vi "data-center-monitor-compare-power-rate.vi"() -> ()   [LabVIEW 2024]
doc: "Demonstrates how to implement advanced power measurement of harmonic parameters on a three-phase electrical power system, such as measurement of harmonic distortion factor, total harmonic distortion, harmonic power, etc. Measurement of harmonic parameters is based on a resampling algorithm."
uses:
  <vilib>/Utility/error.llb/DialogType.ctl
  <vilib>/addons/Electrical Power/Power Measurement/subVIs/ep_Resampled Data.ctl
  <vilib>/DAQmx/read.llb/DAQmx Read (Analog 1D Wfm NChan NSamp).vi
  <extravilib>/ChannelInstances/Tag-bool/Read.vi
  <extravilib>/ChannelInstances/Tag-bool/Write With Abort.vi
  <extravilib>/ChannelInstances/Tag-bool/Read With Abort.vi
  <extravilib>/ChannelInstances/Tag-bool/Instantiate.vi
  <extravilib>/ChannelInstances/Tag-bool/EndpointRead.vi
  <extravilib>/ChannelInstances/Tag-bool/Endpoint.vi
  <vilib>/addons/Electrical Power/Basic/Measurement/Fundamental Vector (N Channels).vi
  <vilib>/DAQmx/miscellaneous.llb/DAQmx Fill In Error Info.vi
  <vilib>/DAQmx/create/channels.llb/DAQmx Create Channel (AI-Voltage-Basic).vi
  <vilib>/DAQmx/create/channels.llb/DAQmx Create Channel (AI-Current-Basic).vi
  <vilib>/DAQmx/configure/timing.llb/DAQmx Timing (Sample Clock).vi
  <resource>/objmgr/daqmx.rc
  <vilib>/addons/Electrical Power/Power Measurement/NI_EP_Power Measurement.lvlib
  <vilib>/addons/Electrical Power/Basic/NI_EP_Basic.lvlib
  <extravilib>/ChannelInstances/Tag-bool.lvlib
panel:
  in  "Display":T1(tab)
  in  "Configuration":enum32{"DAQmx", "Others"}(tab)
  in  "number of samples per channel":i32=10000
  in  "DAQmx sample rate [Hz]":dbl=50000.0 format="%0.2f"
  in  "current channels":tag="current-input/ai0:2"
  in  "maximum current value":dbl=0.002 format="%0.3f"
  in  "minimum current value":dbl=-0.002 format="%0.3f"
  in  "voltage channels":tag="voltage-input/ai0:2"
  in  "maximum voltage value":dbl=300.0 format="%0.2f"
  in  "minimum voltage value":dbl=-300.0 format="%0.2f"
  in  "frequency range [Hz]":cluster{"minimum":dbl, "maximum":dbl}={"minimum"=45.0, "maximum"=65.0}
  in  "samples per cycle":u16=192
  in  "cycles per block":u16=10
  in  "maximum harmonic  order":u16=50
  in  "distortion factor denominator":enum16{"Fundamental value", "Total value"}(ring)
  in  "filter for frequency measurement":T2={"enable filter? (T)"=TRUE, "passband edge frequency [Hz]"=65.0, "passband ripple [dB]"=0.1, "stopband edge frequency [Hz]"=85.0, "stopband attenuation [dB]"=60.0}
  out "Service Rack":cluster{dbl[], dbl[]}[](graph)
  out "PDU":cluster{dbl[], dbl[]}[](graph)
  out "V THD [%]":dbl[](array[numeric]) format="%#_2g"
  out "I THD [%]":dbl[](array[numeric]) format="%#_2g"
  out "Average Frequency [Hz]":dbl format="%#_4g"
  out "Power Usage":T3(graph)
  in  "pause wfm":bool
  out "Time Domain":T4(graph)
  in  "Pause Button":bool
  out "Active Power":waveform(dbl)[](graph)
  out "Voltage Harmonic Spectra":T5(graph)
  out "Current Harmonic Spectra":T5(graph)
  out "voltage total values":dbl[](array[numeric])
  out "voltage THD [%]":dbl[](array[numeric])
  out "voltage harmonic distortion factors [%]":dbl[][](array[numeric])
  out "current THD [%]":dbl[](array[numeric])
  out "total power value":T3
  out "harmonic power values":T6(array[cluster])
  out "power values":T7(array[cluster])
  out "Fundamental Voltage Vectors (Vrms)":cluster{dbl[], dbl[]}[](graph)
  out "Fundamental Current Vectors (Arms)":cluster{dbl[], dbl[]}[](graph)
  out "power history":T3(graph)
  in  "pause-update":bool
  in  "stop":bool
  # "Data Center Power Monitor Demo"
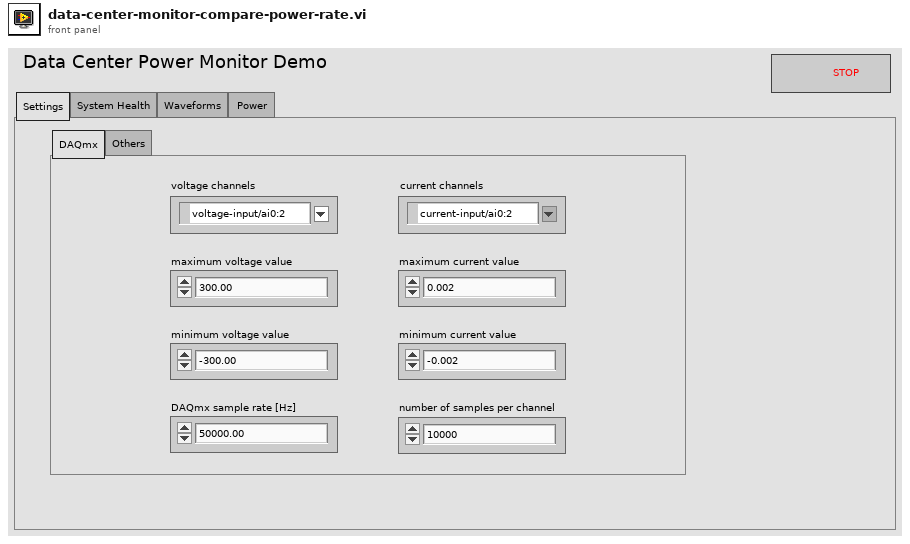
[diagram p1: front panel]
types:
  T1 = enum32{"Settings", "System Health", "Waveforms", "Power ", "V Spectra", "I Spectra", "Basic Parameters", "Harmonic Power", "Phasor", "History"}
  T2 = cluster{"enable filter? (T)":bool, "passband edge frequency [Hz]":dbl, "passband ripple [dB]":dbl, "stopband edge frequency [Hz]":dbl, "stopband attenuation [dB]":dbl}
  T3 = cluster{"active power [W]":dbl, "apparent power [VA]":dbl, "reactive power [VAR]":dbl, "power factor":dbl}
  T4 = cluster{"times [s]":dbl[], "resampled signal":dbl[]}[]
  T5 = cluster{"order 0":dbl, "delta order":dbl, "complex spectrum":dbl[]}[]
  T6 = cluster{"active power [W]":dbl, "apparent power [VA]":dbl, "reactive power [VAR]":dbl, "power factor":dbl}[][]
  T7 = cluster{"active power [W]":dbl, "apparent power [VA]":dbl, "reactive power [VAR]":dbl, "power factor":dbl}[]
  T8 = typedef "NI_EP_Power Measurement.lvlib/ep_Resampled Data.ctl" = cluster{"times [s]":dbl[], "resampled signal":dbl[]}
  T9 = typedef "DialogType.ctl" = u16
  T10 = cluster{"zero crossing times [s]":dbl[], "zero crossings per cycle":u8}
  T11 = typedef "Tag-bool.lvlib/))Channel.ctl" = refnum<queue>
  T12 = cluster{"order 0":dbl, "delta order":dbl, "complex spectrum":cdb[]}[]
  T13 = typedef "NI_EP_Basic.lvlib/basic_Power Value.ctl" = cluster{"active power [W]":dbl, "apparent power [VA]":dbl, "reactive power [VAR]":dbl, "power factor":dbl}
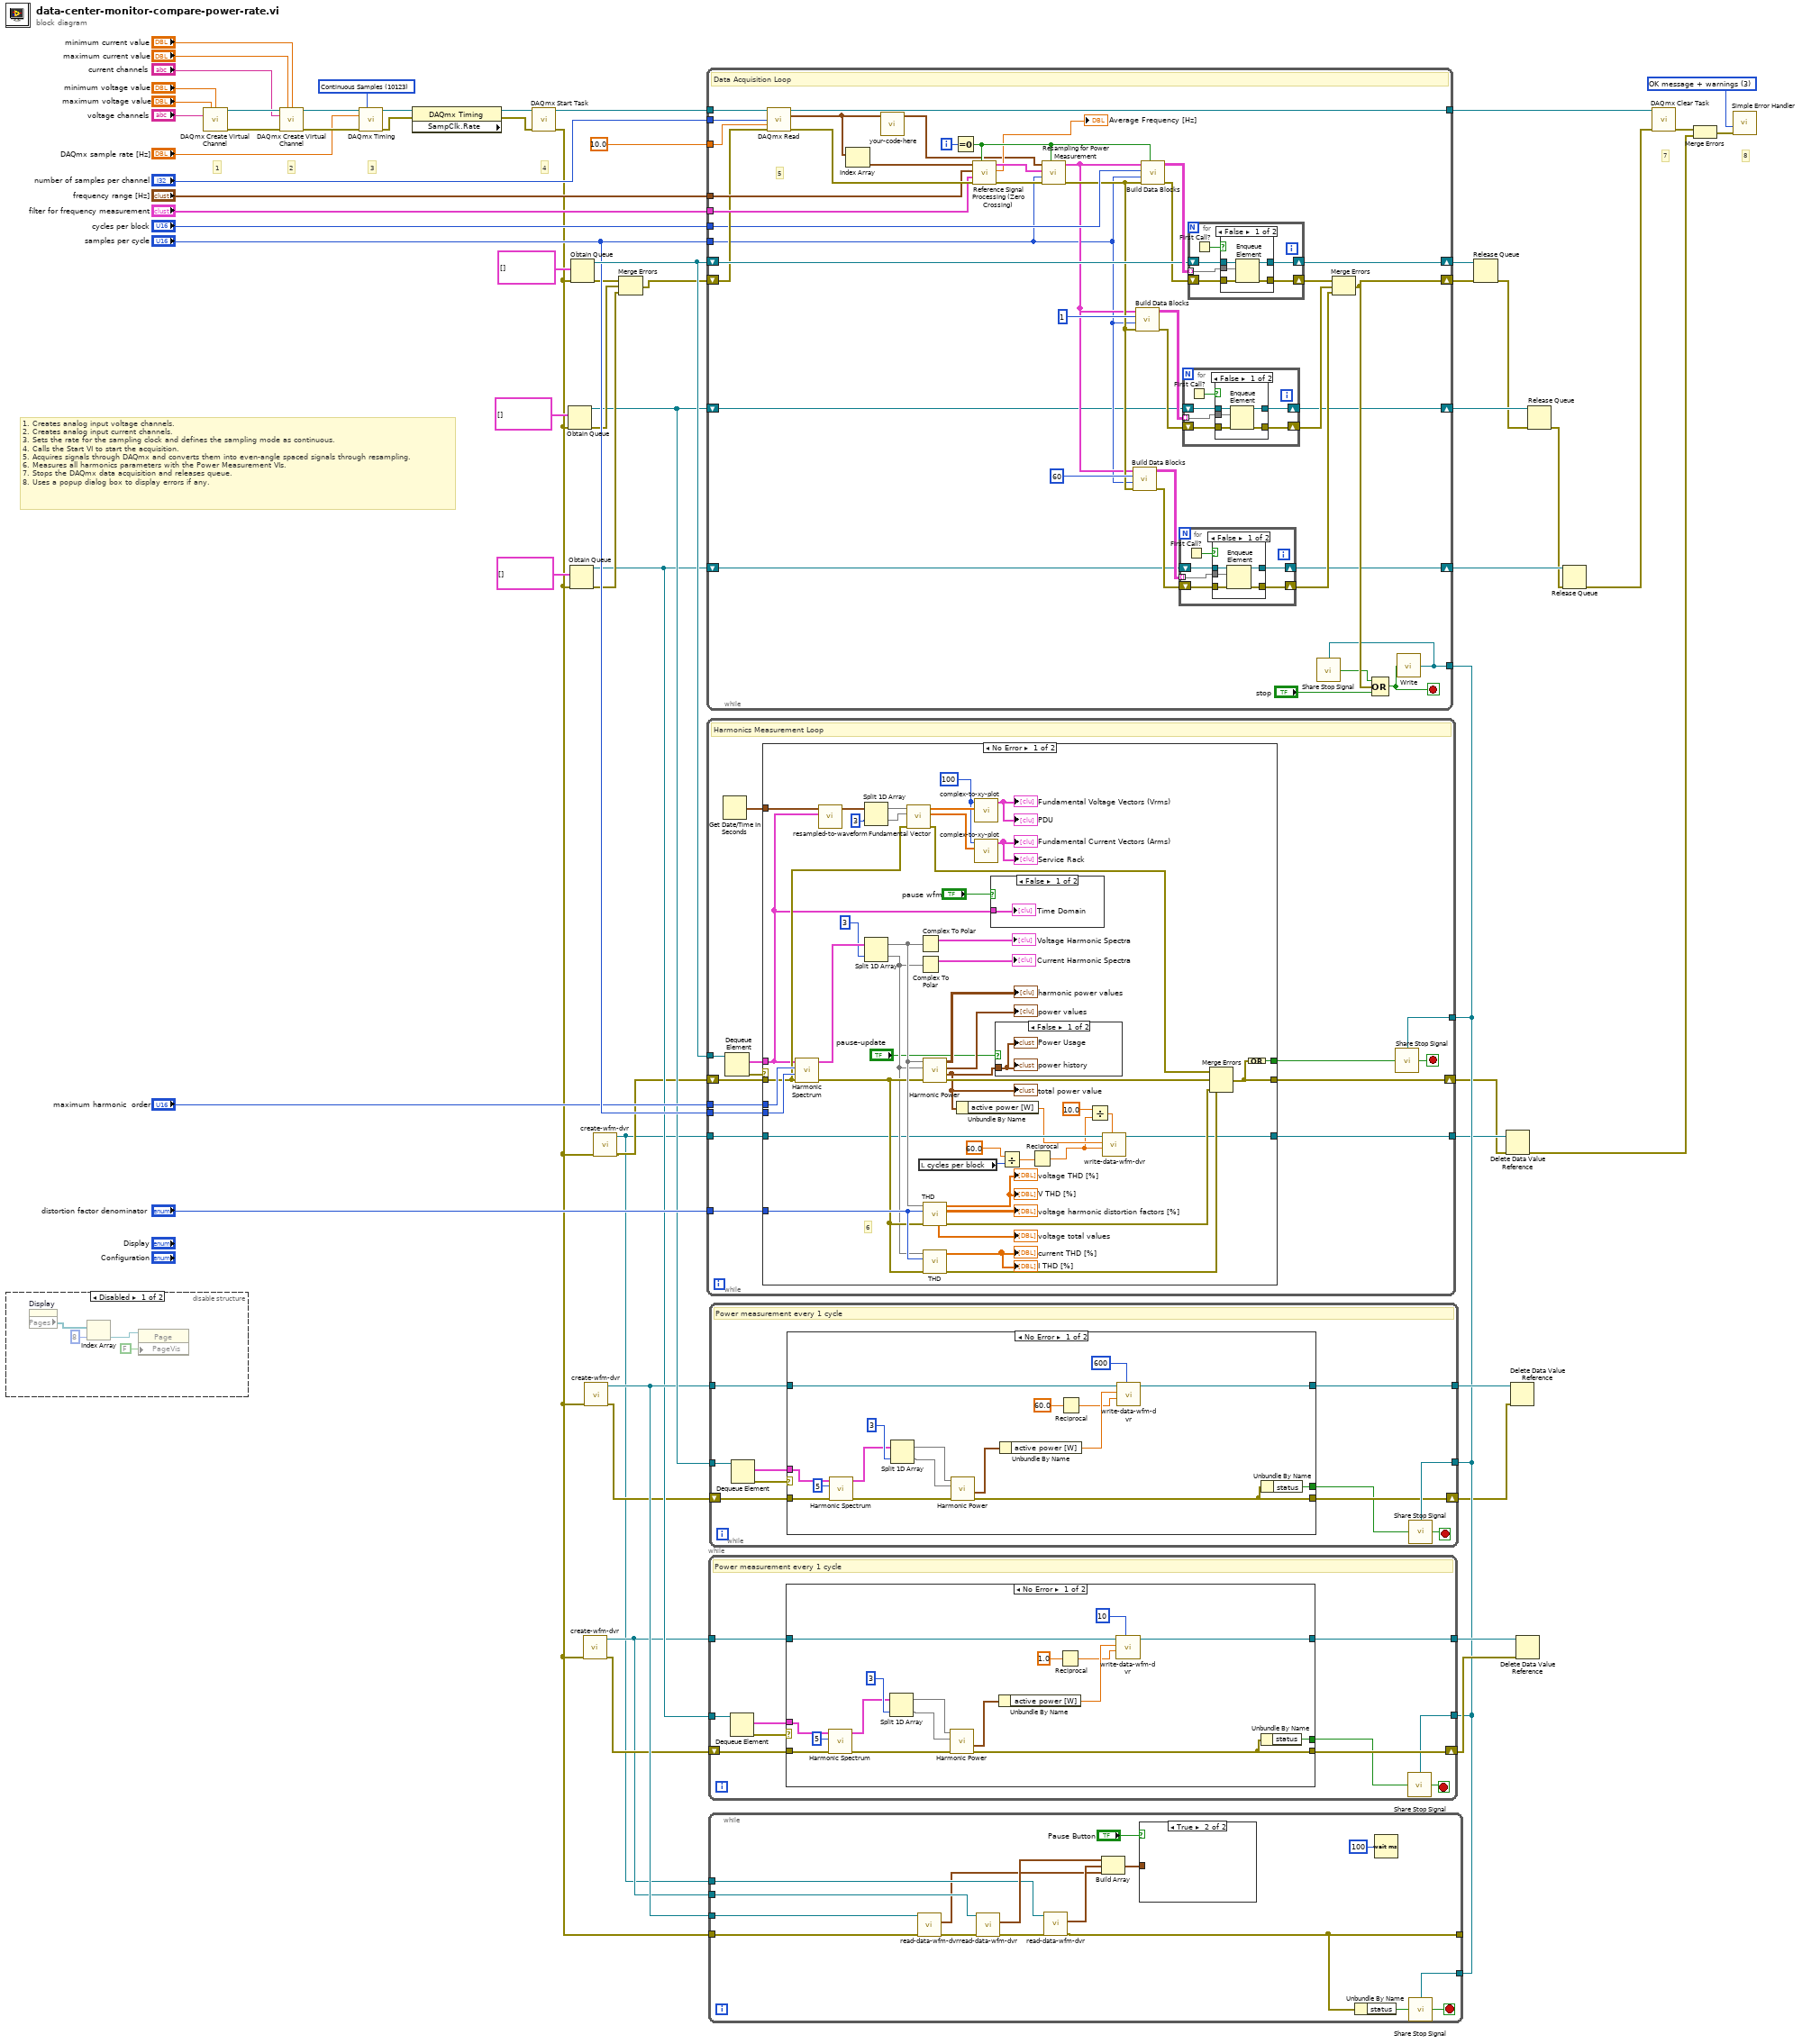
[diagram p0: block diagram]
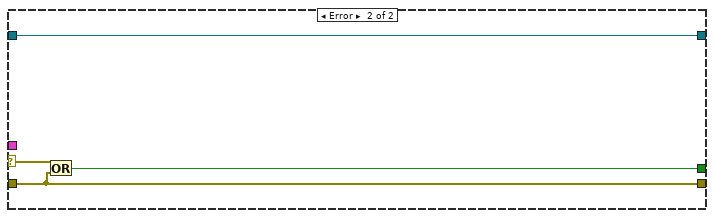
[diagram p3: hidden frame]
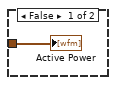
[diagram p4: hidden frame]
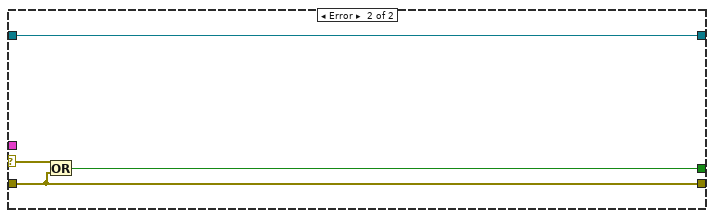
[diagram p5: hidden frame]
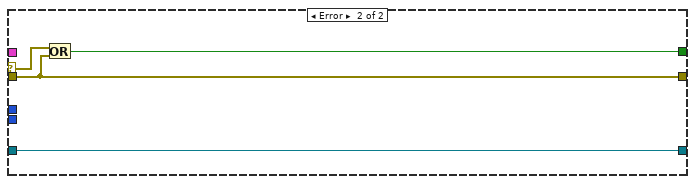
[diagram p8: hidden frame]
diagram:
  w32 = T9 3 items=["no dialog", "OK message", "continue or stop message", "OK message + warnings", "continue/stop + warnings"] ("type of dialog (OK msg:1)")
  w34 = 10123 items=["Finite Samples"=10178, "Continuous Samples"=10123, "Hardware Timed Single Point"=12522] ("sample mode")
  # "8"
  # "7"
  # "1. Creates analog input voltage channels.\n2. Creates analog input current channels.\n3. Sets the rate for the sampling clock and defines the sampling mode as continuous.\n4. Calls the Start VI to start the acquisition.\n5. Acquires signals through DAQmx and converts them into even-angle spaced signals through resampling. \n6. Measures all harmonics parameters with the Power Measurement VIs.\n7.\tStops the DAQmx data acquisition and releases queue.\n8. Uses a popup dialog box to display errors if any."
  # "4"
  # "3"
  # "2"
  # "1"
  n1 = disable-structure shown="Disabled" {
    frame Disabled {
      n2 = property on="Display" class="TabCtl (strict)"() -> ("Pages"=w65:refnum<vi>[])  [unwired: 2 in, 2 out]
      n3 = Index Array(array=w65, index=8) -> (element=w64:refnum<vi>)
      n4 = property class="Page"(reference=w64, "PageVis"=FALSE ("Page Visible")) -> ()  [unwired: 1 in, 2 out]
    }
    frame Enabled {
    }
  }
  n5 = call-poly <vilib>:"DAQmx Create Virtual Channel.vi"("maximum value"="maximum voltage value", "minimum value"="minimum voltage value", "physical channels"="voltage channels") -> ("task out"=w57:refnum<k21>, "error out"=w58:errorcluster)  [unwired: 11 in]
  n6 = call-poly <vilib>:"DAQmx Create Virtual Channel.vi"("task in"=w57, "maximum value"="maximum current value", "minimum value"="minimum current value", "physical channels"="current channels", "error in"=w58) -> ("task out"=w52:refnum<k21>, "error out"=w53:errorcluster)  [unwired: 9 in]
  n7 = call-poly <vilib>:"DAQmx Timing.vi"("task/channels in"=w52, "sample mode"=w34, "rate"="DAQmx sample rate [Hz]", "error in"=w53) -> ("task out"=w46:refnum<k21>, "error out"=w50:errorcluster)  [unwired: 10 in]
  n8 = property class="DAQmx Timing" props=["SampClk.Rate"](reference=w46, error in=w50) -> (reference out=w49:refnum<k21>, error out=w48:errorcluster)  [unwired: 1 out]
  n9 = call <vilib>:"DAQmx Start Task.vi"("task/channels in"=w49, "error in"=w48) -> ("task out"=w47:refnum<k21>, "error out"=w6:errorcluster)  [unwired: 12 in]
  n10 = Obtain Queue(element data type=T8[] [] ("resampled data"), error in (no error)=w6) -> (queue out=w17:refnum<queue>, error out=w24:errorcluster)  [unwired: 3 in, 1 out]
  n11 = Obtain Queue(element data type=T8[] [] ("resampled data"), error in (no error)=w6) -> (queue out=w14:refnum<queue>, error out=w23:errorcluster)  [unwired: 3 in, 1 out]
  n12 = Obtain Queue(element data type=T8[] [] ("resampled data"), error in (no error)=w6) -> (queue out=w39:refnum<queue>, error out=w26:errorcluster)  [unwired: 3 in, 1 out]
  n13 = call "create-wfm-dvr.vi"("error in (no error)"=w6) -> ("error out"=w12:errorcluster, "wfm dvr"=w11:refnum<data-value>)  [unwired: 9 in]
  n14 = call "create-wfm-dvr.vi"("error in (no error)"=w6) -> ("error out"=w13:errorcluster, "wfm dvr"=w15:refnum<data-value>)  [unwired: 9 in]
  n15 = call "create-wfm-dvr.vi"("error in (no error)"=w6) -> ("error out"=w5:errorcluster, "wfm dvr"=w1:refnum<data-value>)  [unwired: 9 in]
  n16 = Merge Errors(w26, w24, w23) -> (w25:errorcluster)
  n17 = while {
    tunnel: "number of samples per channel" -> [w106]
    tunnel: w47 -> [w107]
    tunnel: [w105] -> w44
    tunnel: "frequency range [Hz]" -> [w101]
    tunnel: "filter for frequency measurement" -> [w100]
    shift-right: [w93] -> w41
    shift-left: w39 -> [w95]
    shift-right: [w75] -> w30
    shift-left: w25 -> [w94]
    tunnel: "samples per cycle" -> [w77]
    tunnel: "cycles per block" -> [w92]
    tunnel: 10.0 ("timeout") -> [w90]
    shift-right: [w71] -> w22
    shift-left: w17 -> [w72]
    shift-right: [w69] -> w20
    shift-left: w14 -> [w70]
    tunnel: [w67] -> w8
    i -> [w103]
    stop <- w68 stop-if-true
    # "5"
    # "Data Acquisition Loop"
    n18 = call-poly <vilib>:"DAQmx Read.vi"("task/channels in"=w107, "number of samples per channel"=w106, "timeout"=w90, "error in"=w94) -> ("task out"=w105:refnum<k21>, "data"=w87:waveform(dbl)[], "error out"=w104:errorcluster)  [unwired: 9 in]
    n19 = Index Array(array=w87) -> (element=w102:waveform(dbl))  [unwired: 1 in]
    n20 = call "your-code-here.vi"("data in"=w87) -> ("data out"=w86:waveform(dbl)[])  [unwired: 10 in]
    n21 = Equal To 0?(x=w103) -> (x = 0?=w97:bool)
    n22 = call <vilib>:"Reference Signal Processing (Zero Crossing).vi"("reset? (F)"=w97, "error in (no error)"=w104, "filter for frequency measurement"=w100, "frequency range [Hz]"=w101, "reference signal"=w102) -> ("error out"=w99:errorcluster, "average frequency [Hz]"=→"Average Frequency [Hz]":dbl, "zero crossing information"=w98:T10)  [unwired: 3 in, 1 out]
    n23 = call <vilib>:"Resampling for Power Measurement.vi"("reset? (F)"=w97, "error in (no error)"=w99, "samples per cycle (192)"=w77, "trigger information"=w98, "data in"=w86) -> ("error out"=w79:errorcluster, "resampled data"=w78:T8[])  [unwired: 5 in]
    n24 = call <vilib>:"Build Data Blocks.vi"("error in (no error)"=w79, "samples per cycle (192)"=w77, "cycles per block (10)"=u16 60, "resampled data"=w78) -> ("error out"=w81:errorcluster, "data blocks"=w80:T8[][])  [unwired: 6 in]
    n25 = call <vilib>:"Build Data Blocks.vi"("error in (no error)"=w79, "samples per cycle (192)"=w77, "cycles per block (10)"=u16 1, "resampled data"=w78) -> ("error out"=w84:errorcluster, "data blocks"=w85:T8[][])  [unwired: 6 in]
    n26 = call <vilib>:"Build Data Blocks.vi"("reset? (F)"=w97, "error in (no error)"=w79, "samples per cycle (192)"=w77, "cycles per block (10)"=w92, "resampled data"=w78) -> ("error out"=w89:errorcluster, "data blocks"=w96:T8[][])  [unwired: 5 in]
    n27 = for {
      shift-right: [w111] -> w69
      shift-left: w70 -> [w112]
      shift-right: [w113] -> w73
      shift-left: w81 -> [w110]
      tunnel: w80 -> [w109] mode=indexing
      n28 = First Call?() -> (First Call?: T/F=w108:bool)
      n29 = case shown="False" w108 {
        tunnel: [w118 w119] -> w113
        tunnel: w112 -> [w117 w120]
        tunnel: [w116 w120] -> w111
        tunnel: w110 -> [w115 w119]
        tunnel: w109 -> [w114 _]
        frame False {
          n30 = Enqueue Element(queue=w117, element=w114, error in (no error)=w115) -> (queue out=w116:refnum<queue>, error out=w118:errorcluster)  [unwired: 1 in, 1 out]
        }
        frame True {
        }
      }
    }
    n31 = for {
      shift-right: [w124] -> w71
      shift-left: w72 -> [w125]
      shift-right: [w126] -> w74
      shift-left: w84 -> [w123]
      tunnel: w85 -> [w122] mode=indexing
      n32 = First Call?() -> (First Call?: T/F=w121:bool)
      n33 = case shown="False" w121 {
        tunnel: [w131 w132] -> w126
        tunnel: w125 -> [w130 w133]
        tunnel: [w129 w133] -> w124
        tunnel: w123 -> [w128 w132]
        tunnel: w122 -> [w127 _]
        frame False {
          n34 = Enqueue Element(queue=w130, element=w127, error in (no error)=w128) -> (queue out=w129:refnum<queue>, error out=w131:errorcluster)  [unwired: 1 in, 1 out]
        }
        frame True {
        }
      }
    }
    n35 = for {
      shift-right: [w137] -> w93
      shift-left: w95 -> [w138]
      shift-right: [w139] -> w76
      shift-left: w89 -> [w136]
      tunnel: w96 -> [w135] mode=indexing
      n36 = First Call?() -> (First Call?: T/F=w134:bool)
      n37 = case shown="False" w134 {
        tunnel: [w144 w145] -> w139
        tunnel: w138 -> [w143 w146]
        tunnel: [w142 w146] -> w137
        tunnel: w136 -> [w141 w145]
        tunnel: w135 -> [w140 _]
        frame False {
          n38 = Enqueue Element(queue=w143, element=w140, error in (no error)=w141) -> (queue out=w142:refnum<queue>, error out=w144:errorcluster)  [unwired: 1 in, 1 out]
        }
        frame True {
        }
      }
    }
    n39 = Merge Errors(w76, w74, w73) -> (w75:errorcluster)
    n40 = call <vilib>:"Share Stop Signal.vi"("channel"=w67) -> ("stop"=w66:bool)  [unwired: 1 in]
    n41 = Compound Arithmetic op=OR(w66, w75, "stop") -> (w68:bool)
    n42 = call <extravilib>:"Write.vi"("element"=w68) -> ("channel"=w67:T11)  [unwired: 1 out]
  }
  n43 = while {
    shift-right: [w152] -> w3
    shift-left: w5 -> [w155]
    tunnel: w39 -> [w160]
    tunnel: "samples per cycle" -> [w158]
    tunnel: "maximum harmonic  order" -> [w157]
    tunnel: "distortion factor denominator" -> [w156]
    tunnel: w8 -> [w149]
    tunnel: w1 -> [w148]
    tunnel: [w147] -> w4
    stop <- w153 stop-if-true
    # "Harmonics Measurement Loop"
    n44 = Get Date/Time In Seconds() -> (seconds since 1Jan1904=w150:timestamp)
    n45 = Dequeue Element(queue=w160) -> (element=w159:T8[], error out=w154:errorcluster)  [unwired: 2 in, 2 out]
    n46 = case shown="No Error" w154 {
      selector: w154 -> [_ w212]
      tunnel: w159 -> [w165 _]
      tunnel: w158 -> [w206 _]
      tunnel: w157 -> [w205 _]
      tunnel: w155 -> [w183 w211]
      tunnel: [w198 w211] -> w152
      tunnel: w156 -> [w202 _]
      tunnel: [w193 w210] -> w151
      tunnel: w150 -> [w191 _]
      tunnel: w148 -> [w174 w209]
      tunnel: [w173 w209] -> w147
      frame No Error {
        w184 = 100
        # "6"
        n47 = call <vilib>:"Harmonic Spectrum.vi"("error in (no error)"=w183, "samples per cycle (192)"=w206, "maximum harmonic order (50)"=w205, "resampled data"=w165) -> ("error out"=w194:errorcluster, "harmonic spectra"=w204:T12)  [unwired: 6 in]
        n48 = call "resampled-to-waveform.vi"("resampled data"=w165, "current-timestamp"=w191) -> ("waveform data"=w189:waveform(dbl)[])  [unwired: 9 in]
        n49 = Split 1D Array(array=w189, index=3) -> (first subarray=w188:waveform(dbl)[], second subarray=w187:waveform(dbl)[])
        n50 = Split 1D Array(array=w204, index=3) -> (first subarray=w203:T12, second subarray=w180:T12)
        n51 = call-poly <vilib>:"Fundamental Vector.vi"("error in (no error)"=w183, "current waveforms"=w187, "voltage waveforms"=w188) -> ("error out"=w182:errorcluster, "current fundamental vectors"=w185:cdb[], "voltage fundamental vectors"=w186:cdb[])  [unwired: 5 in, 1 out]
        n52 = Complex To Polar(r * e^(i*theta)=w203) -> (r=→"Voltage Harmonic Spectra":T5)  [unwired: 1 out]
        n53 = Complex To Polar(r * e^(i*theta)=w180) -> (r=→"Current Harmonic Spectra":T5)  [unwired: 1 out]
        n54 = local read "cycles per block"() -> (w171:u16)
        n55 = call <vilib>:"Harmonic Power.vi"("error in (no error)"=w194, "current spectra"=w180, "voltage spectra"=w203) -> ("error out"=w199:errorcluster, "total power value"=w162:T13, "power values"=→"power values":T13[], "harmonic power values"=→"harmonic power values":T13[][])  [unwired: 5 in]
        "total power value" <- w162
        n56 = call <vilib>:"THD.vi"("error in (no error)"=w194, "distortion factor denominator"=w202, "harmonic spectra"=w203) -> ("error out"=w195:errorcluster, "harmonic distortion factors [%]"=→"voltage harmonic distortion factors [%]":dbl[][], "THD [%]"=→"voltage THD [%]" →"V THD [%]":dbl[], "total values"=→"voltage total values":dbl[])  [unwired: 5 in]
        n57 = call <vilib>:"THD.vi"("error in (no error)"=w194, "distortion factor denominator"=w202, "harmonic spectra"=w180) -> ("error out"=w197:errorcluster, "THD [%]"=→"current THD [%]" →"I THD [%]":dbl[])  [unwired: 5 in, 2 out]
        n58 = Unbundle By Name(w162) -> ("active power [W]"=w172:dbl)
        n59 = call "complex-to-xy-plot.vi"("complex-vector"=w186, "number-of-points"=w184) -> ("xy-plot-output"=→"Fundamental Voltage Vectors (Vrms)" →"PDU":cluster{dbl[], dbl[]}[])  [unwired: 9 in]
        n60 = call "complex-to-xy-plot.vi"("complex-vector"=w185, "number-of-points"=w184) -> ("xy-plot-output"=→"Fundamental Current Vectors (Arms)" →"Service Rack":cluster{dbl[], dbl[]}[])  [unwired: 9 in]
        n61 = case shown="False" "pause wfm" {
          tunnel: w165 -> [w207 _]
          frame False {
            "Time Domain" <- w207
          }
          frame True {
          }
        }
        n62 = case shown="False" "pause-update" {
          tunnel: w162 -> [w208 _]
          frame False {
            "power history" <- w208
            "Power Usage" <- w208
          }
          frame True {
          }
        }
        n63 = Divide(x=60.0, y=w171) -> (x/y=w169:dbl)
        n64 = Reciprocal(x=w169) -> (1/x=w167:dbl)
        n65 = Divide(x=10.0, y=w167) -> (x/y=w166:dbl)
        n66 = call "write-data-wfm-dvr.vi"("wfm size"=w166, "dt"=w167, "data"=w172, "wfm dvr"=w174) -> ("wfm dvr"=w173:refnum<data-value>)  [unwired: 6 in, 1 out]
        n67 = Merge Errors(w182, w199, w195, w197) -> (w198:errorcluster)
        n68 = Compound Arithmetic op=OR(w198) -> (w193:bool)
      }
      frame Error {
        n69 = Or(x=w212, y=w211) -> (x .or. y?=w210:bool)
      }
    }
    n70 = call <vilib>:"Share Stop Signal.vi"("set stop (F)"=w151, "channel"=w149) -> ("stop"=w153:bool)
  }
  n71 = while {
    shift-right: [w217] -> w9
    shift-left: w12 -> [w221]
    tunnel: w14 -> [w222]
    tunnel: w8 -> [w213]
    tunnel: w11 -> [w215]
    tunnel: [w214] -> w10
    stop <- w218 stop-if-true
    # "Power measurement every 1 cycle"
    n72 = Dequeue Element(queue=w222) -> (element=w219:T8[], error out=w220:errorcluster)  [unwired: 2 in, 2 out]
    n73 = case shown="No Error" w220 {
      selector: w220 -> [_ w243]
      tunnel: w221 -> [w238 w242]
      tunnel: w219 -> [w235 _]
      tunnel: [w228 w242] -> w217
      tunnel: [w239 w241] -> w216
      tunnel: w215 -> [w227 w240]
      tunnel: [w226 w240] -> w214
      frame No Error {
        n74 = call <vilib>:"Harmonic Spectrum.vi"("error in (no error)"=w238, "maximum harmonic order (50)"=u16 5, "resampled data"=w235) -> ("error out"=w234:errorcluster, "harmonic spectra"=w236:T12)  [unwired: 7 in]
        n75 = Split 1D Array(array=w236, index=3) -> (first subarray=w233:T12, second subarray=w232:T12)
        n76 = call <vilib>:"Harmonic Power.vi"("error in (no error)"=w234, "current spectra"=w232, "voltage spectra"=w233) -> ("error out"=w228:errorcluster, "total power value"=w231:T13)  [unwired: 5 in, 2 out]
        n77 = Unbundle By Name(w231) -> ("active power [W]"=w225:dbl)
        n78 = Reciprocal(x=1.0) -> (1/x=w224:dbl)
        n79 = call "write-data-wfm-dvr.vi"("wfm size"=10, "dt"=w224, "data"=w225, "wfm dvr"=w227) -> ("wfm dvr"=w226:refnum<data-value>)  [unwired: 6 in, 1 out]
        n80 = Unbundle By Name(w228) -> ("status"=w239:bool)
      }
      frame Error {
        n81 = Or(x=w243, y=w242) -> (x .or. y?=w241:bool)
      }
    }
    n82 = call <vilib>:"Share Stop Signal.vi"("set stop (F)"=w216, "channel"=w213) -> ("stop"=w218:bool)
  }
  n83 = while {
    tunnel: w6 -> [w256]
    tunnel: w8 -> [w259]
    tunnel: [w249] -> _
    tunnel: w15 -> [w255]
    tunnel: w11 -> [w254]
    tunnel: w1 -> [w247]
    stop <- w258 stop-if-true
    n84 = call "read-data-wfm-dvr.vi"("error in (no error)"=w256, "wfm dvr"=w255) -> ("error out"=w253:errorcluster, "Waveform"=w245:waveform(dbl))  [unwired: 8 in]
    n85 = call "read-data-wfm-dvr.vi"("error in (no error)"=w253, "wfm dvr"=w254) -> ("error out"=w250:errorcluster, "Waveform"=w252:waveform(dbl))  [unwired: 8 in]
    n86 = call "read-data-wfm-dvr.vi"("error in (no error)"=w250, "wfm dvr"=w247) -> ("error out"=w249:errorcluster, "Waveform"=w248:waveform(dbl))  [unwired: 8 in]
    n87 = Build Array(w252, w248, w245) -> (w251:waveform(dbl)[])
    n88 = case shown="True" "Pause Button" {
      tunnel: w251 -> [w260 _]
      frame False {
        "Active Power" <- w260
      }
      frame True {
      }
    }
    n89 = Unbundle By Name(w249) -> ("status"=w257:bool)
    n90 = Wait (ms)(milliseconds to wait=u32 100) -> ()  [unwired: 1 out]
    n91 = call <vilib>:"Share Stop Signal.vi"("set stop (F)"=w257, "channel"=w259) -> ("stop"=w258:bool)
  }
  n92 = while {
    shift-right: [w264] -> w7
    shift-left: w13 -> [w269]
    tunnel: w17 -> [w270]
    tunnel: w8 -> [w265]
    tunnel: w15 -> [w262]
    tunnel: [w261] -> w16
    stop <- w266 stop-if-true
    # "Power measurement every 1 cycle"
    n93 = Dequeue Element(queue=w270) -> (element=w267:T8[], error out=w268:errorcluster)  [unwired: 2 in, 2 out]
    n94 = case shown="No Error" w268 {
      selector: w268 -> [_ w291]
      tunnel: w269 -> [w286 w290]
      tunnel: w267 -> [w283 _]
      tunnel: [w276 w290] -> w264
      tunnel: [w287 w289] -> w263
      tunnel: w262 -> [w275 w288]
      tunnel: [w274 w288] -> w261
      frame No Error {
        n95 = call <vilib>:"Harmonic Spectrum.vi"("error in (no error)"=w286, "maximum harmonic order (50)"=u16 5, "resampled data"=w283) -> ("error out"=w282:errorcluster, "harmonic spectra"=w284:T12)  [unwired: 7 in]
        n96 = Split 1D Array(array=w284, index=3) -> (first subarray=w281:T12, second subarray=w280:T12)
        n97 = call <vilib>:"Harmonic Power.vi"("error in (no error)"=w282, "current spectra"=w280, "voltage spectra"=w281) -> ("error out"=w276:errorcluster, "total power value"=w279:T13)  [unwired: 5 in, 2 out]
        n98 = Unbundle By Name(w279) -> ("active power [W]"=w273:dbl)
        n99 = Reciprocal(x=60.0) -> (1/x=w272:dbl)
        n100 = call "write-data-wfm-dvr.vi"("wfm size"=600, "dt"=w272, "data"=w273, "wfm dvr"=w275) -> ("wfm dvr"=w274:refnum<data-value>)  [unwired: 6 in, 1 out]
        n101 = Unbundle By Name(w276) -> ("status"=w287:bool)
      }
      frame Error {
        n102 = Or(x=w291, y=w290) -> (x .or. y?=w289:bool)
      }
    }
    n103 = call <vilib>:"Share Stop Signal.vi"("set stop (F)"=w263, "channel"=w265) -> ("stop"=w266:bool)
  }
  n104 = Release Queue(queue=w41, error in (no error)=w30) -> (error out=w21:errorcluster)  [unwired: 1 in, 2 out]
  n105 = Delete Data Value Reference(data value reference=w4, error in=w3) -> (error out=w2:errorcluster)  [unwired: 1 out]
  n106 = Delete Data Value Reference(data value reference=w16, error in=w7) -> ()  [unwired: 2 out]
  n107 = Delete Data Value Reference(data value reference=w10, error in=w9) -> ()  [unwired: 2 out]
  n108 = Release Queue(queue=w22, error in (no error)=w21) -> (error out=w19:errorcluster)  [unwired: 1 in, 2 out]
  n109 = Release Queue(queue=w20, error in (no error)=w19) -> (error out=w18:errorcluster)  [unwired: 1 in, 2 out]
  n110 = call <vilib>:"DAQmx Clear Task.vi"("task in"=w44, "error in"=w18) -> ("error out"=w29:errorcluster)  [unwired: 13 in]
  n111 = Merge Errors(w29, w2) -> (w35:errorcluster)
  n112 = call <vilib>:"Simple Error Handler.vi"("type of dialog (OK msg:1)"=w32, "error in (no error)"=w35) -> ()  [unwired: 3 in, 5 out]
